vi "Autoscale.vi"(8 "error in (no error)":errorcluster, 11 "MSOX6004 in":refnum<class "MSOX6004.lvclass">) -> (0 "error out":errorcluster, 3 "MSOX6004 out":refnum<class "MSOX6004.lvclass">)   [LabVIEW 2018, in "MSOX6004.lvlib" / "MSOX6004.lvclass"]
doc: "This Override method is used to call the Oscope instrument Autoscale function."
uses:
  MSOX6004.lvclass
  MSOX6004.lvclass/MSOX6004.ctl
  <instrlib>/Keysight InfiniiVision/Keysight InfiniiVision.lvlib
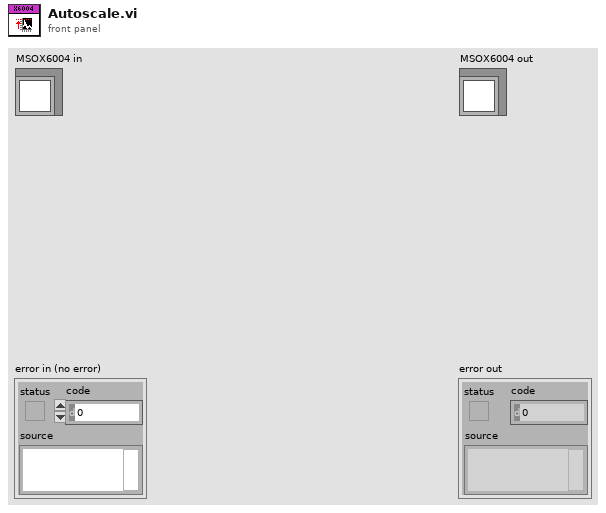
[diagram p1: front panel]
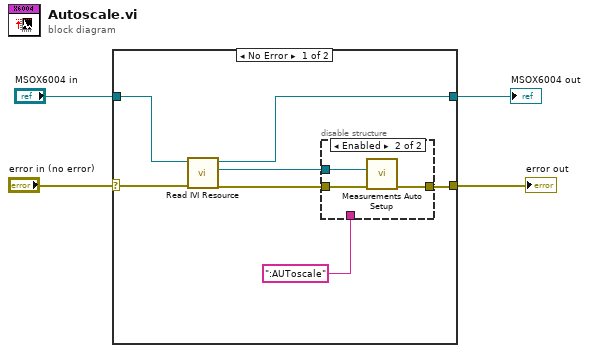
[diagram p0: block diagram]
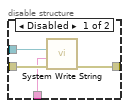
[diagram p2: hidden frame]
diagram:
  n1 = case shown="No Error" "error in (no error)" {
    selector: "error in (no error)" -> [w11 w20]
    tunnel: [w7 w20] -> w3
    tunnel: [w9 w19] -> w2
    tunnel: "MSOX6004 in" -> [w10 w19]
    frame No Error {
      n2 = call "Read IVI Resource.vi"("error in (no error)"=w11, "MSOX6004 in"=w10) -> ("error out"=w8:errorcluster, "IVI Resource"=w5:refnum<k15>, "MSOX6004 out"=w9:refnum<class "MSOX6004.lvclass">)  [unwired: 7 in]
      n3 = disable-structure shown="Enabled" {
        disable-tunnel: w8 -> [w15 w17]
        disable-tunnel: [w14 w16] -> w7
        disable-tunnel: ":AUToscale" ("Data") -> [w13 _]
        disable-tunnel: w5 -> [w12 w18]
        frame Disabled {
          n4 = call <instrlib>:"System Write String.vi"("error in (no error)"=w15, "Data"=w13, "instrument handle"=w12) -> ("error out"=w14:errorcluster)  [unwired: 7 in, 1 out]
        }
        frame Enabled {
          n5 = call <instrlib>:"Measurements Auto Setup.vi"("error in (no error)"=w17, "instrument handle"=w18) -> ("error out"=w16:errorcluster)  [unwired: 8 in, 1 out]
        }
      }
    }
    frame Error {
    }
  }
  "error out" <- w3
  "MSOX6004 out" <- w2
